vi "Phase Space Density.vi"(8 "Trap Frequencies":T1, 9 "Temperature (K) y":dbl format="%#_6p", 10 "Temperature (K) x":dbl format="%#_6p", 11 "Number":dbl) -> (3 "Phase Space Density":dbl format="%#_3e")   [LabVIEW 2016]
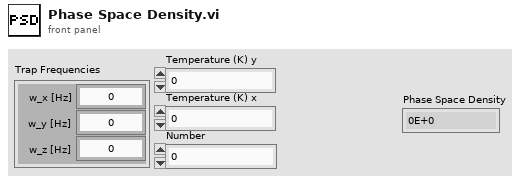
[diagram p1: front panel]
types:
  T1 = cluster{"w_x [Hz]":dbl, "w_y [Hz]":dbl, "w_z [Hz]":dbl}
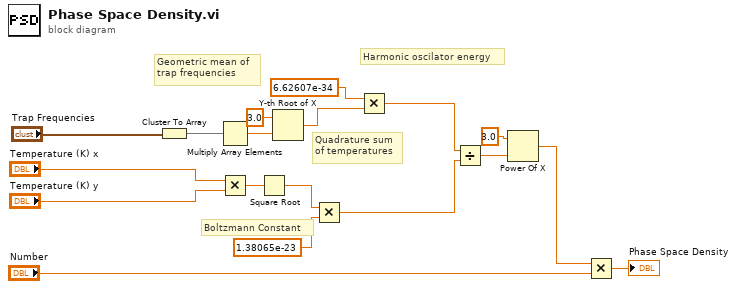
[diagram p0: block diagram]
diagram:
  # "Quadrature sum\nof temperatures"
  # "Boltzmann Constant"
  # "Geometric mean of\ntrap frequencies"
  # "Harmonic oscilator energy"
  n1 = Cluster To Array(cluster="Trap Frequencies") -> (array=w17:dbl[])
  n2 = Multiply Array Elements(1:w17) -> (0:w9:dbl)
  n3 = Multiply(x="Temperature (K) x", y="Temperature (K) y") -> (x*y=w11:dbl)
  n4 = Square Root(x=w11) -> (sqrt(x)=w10:dbl)
  n5 = Y-th Root of X(1:w9, 2:3.0 ("y")) -> (0:w15:dbl)
  n6 = Multiply(x=w10, y=1.38065e-23) -> (x*y=w13:dbl)
  n7 = Multiply(x=6.62607e-34, y=w15) -> (x*y=w14:dbl)
  n8 = Divide(x=w14, y=w13) -> (x/y=w6:dbl)
  n9 = Power Of X(1:w6, 2:3.0 ("y")) -> (0:w5:dbl)
  n10 = Multiply(x=w5, y="Number") -> (x*y=→"Phase Space Density":dbl)
